vi "Go to Idle.vi"(8 "error in (no error)":errorcluster, 11 "Chef State in":refnum<class "Chef State.lvclass">) -> (0 "error out":errorcluster, 3 "Chef State out":refnum<class "State Actor.lvclass">)   [LabVIEW 2024, in "Chef State.lvlib" / "Chef State.lvclass"]
uses:
  Chef State.lvclass
  Chef State.lvclass/Chef State.ctl
  <vilib>/ni/Actors/State Actor/State Actor/State Actor.lvclass
  Idle/Idle.lvclass
  C:/Program Files/National Instruments/LabVIEW 2024/vi.lib/ni/Actors/State Actor/State Actor/State Actor.lvclass
  C:/Program Files/National Instruments/LabVIEW 2024/vi.lib/ActorFramework/Actor/Actor.lvclass
  G:/Leveling/LabVIEW/Learning/Actor Framework/Actor State Machine Learning/Chef State/Chef State/Chef State.lvclass
  G:/Leveling/LabVIEW/Learning/Actor Framework/Actor State Machine Learning/Chef State/Idle/Idle.lvclass
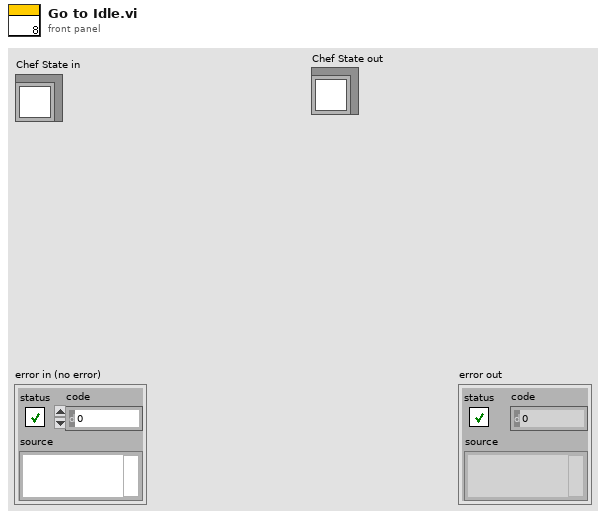
[diagram p1: front panel]
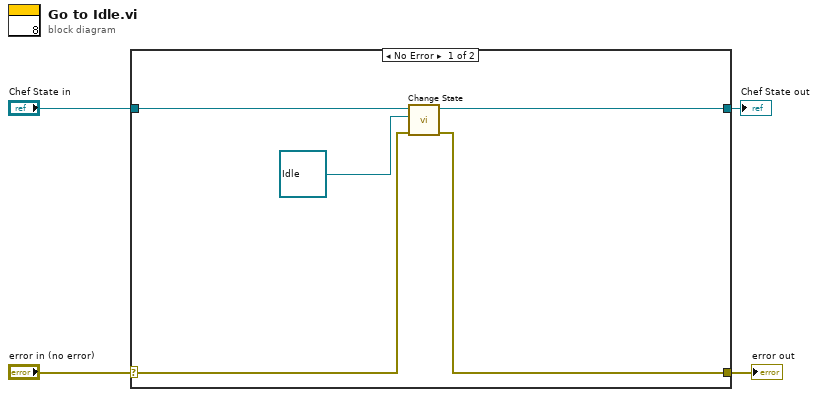
[diagram p0: block diagram]
diagram:
  n1 = case shown="No Error" "error in (no error)" {
    selector: "error in (no error)" -> [w9 w11]
    tunnel: [w8 w11] -> w3
    tunnel: [w6 w10] -> w1
    tunnel: "Chef State in" -> [w7 w10]
    frame No Error {
      n2 = call <vilib>:"Change State.vi"("error in (no error)"=w9, "New State in"=refnum<class "Idle.lvclass"> refnum ("Chef State.lvlib:Idle.lvclass"), "State in"=w7) -> ("error out"=w8:errorcluster, "State out"=w6:refnum<class "State Actor.lvclass">)  [unwired: 7 in]
    }
    frame Error {
    }
  }
  "error out" <- w3
  "Chef State out" <- w1
